vi "Analog Read N Chans.vi"(7 "Analog Ref Override":dbl, 8 "Error In":errorcluster, 10 "AI Channel(s)":u8[](array[numeric]), 11 "LINX Resource":T1) -> (0 "Error Out":errorcluster, 1 "AI Ref":dbl, 2 "Voltages":dbl[](array[numeric]), 3 "LINX Resource":T1)   [LabVIEW 2013, in "LVH-LINX.lvlib"]
doc: "Read the values of the specified analog input channels."
uses:
  <vilib>/LabVIEW Hacker/LINX/LVH-LINX.lvlib
  <vilib>/LabVIEW Hacker/LINX/Private/Type Defs/LINX Ref.ctl
  <vilib>/LabVIEW Hacker/LINX/Private/Type Defs/Platform.ctl
  <vilib>/LabVIEW Hacker/LINX/Private/Type Defs/Interface.ctl
  <vilib>/LabVIEW Hacker/LINX/Private/Device/Type Defs/LINX Device Config.ctl
  <vilib>/LabVIEW Hacker/LINX/Private/Device/Type Defs/TCP Config.ctl
  <vilib>/LabVIEW Hacker/LINX/Private/Type Defs/Device Family.ctl
  <vilib>/LabVIEW Hacker/LINX/Private/Type Defs/Peripheral.ctl
  <vilib>/LabVIEW Hacker/LINX/Private/Device/Device.lvlib
  <vilib>/LabVIEW Hacker/LINX/Private/myRIO/myRIO.lvlib
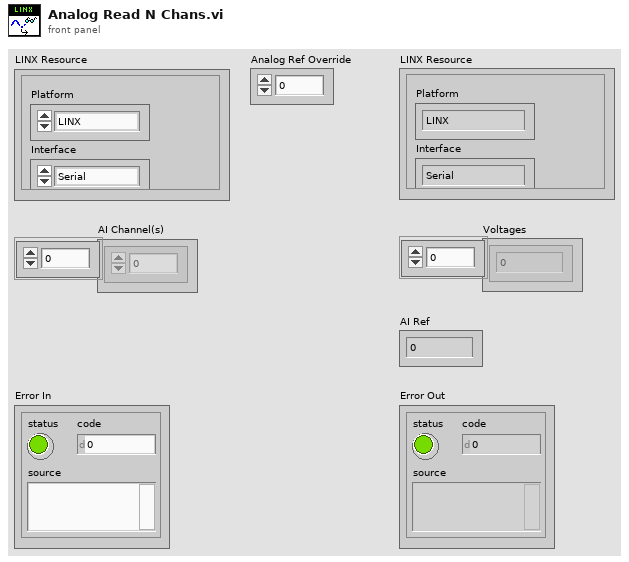
[diagram p1: front panel]
types:
  T1 = typedef "LVH-LINX.lvlib/LINX Ref.ctl" = cluster{"Platform":T2, "Interface":T3, "LINX Device Config":T4}
  T2 = typedef "LVH-LINX.lvlib/Platform.ctl" = enum16{"LINX", "myRIO"}
  T3 = typedef "LVH-LINX.lvlib/Interface.ctl" = enum16{"Serial", "TCP"}
  T4 = typedef "LVH-LINX.lvlib/Device.lvlib/LINX Device Config.ctl" = cluster{"Interface":T3, "COM Port":refnum<visa-resource-name>, "TCP Configuration":T5, "Device Family":T6, "Device ID":u8, "Device Name":string, "TCP Ref":refnum<k5>}
  T5 = typedef "LVH-LINX.lvlib/Device.lvlib/TCP Config.ctl" = cluster{"IP Address":string, "Port":u16}
  T6 = typedef "LVH-LINX.lvlib/Device Family.ctl" = enum8{"National Instruments", "Digilent", "Arduino"}
  T7 = typedef "LVH-LINX.lvlib/Peripheral.ctl" = enum8{"DI", "DO", "AI", "AO", "PWM", "QE", "UART", "I2C", "SPI", "CAN"}
  T8 = typedef "AI.lvlib/AI Reference.ctl" = cluster{"myRIO Reference":T9, "AI Channels List":T13, "AI Scaling Constants List":T15}
  T9 = typedef "myRIO Generic Hardware Reference.ctl" = cluster{"myRIO Model":T10, "myRIO Hardware Reference":T11}
  T10 = typedef "Hardware Version Enum.ctl" = enum16{"Unknown", "myRIO-1900", "myRIO-1950"}
  T11 = typedef "myRIO v1.0 Reference.ctl" = cluster{"Generic FPGA Reference":T12, "Allow multiple opens":bool}
  T12 = typedef "Generic FPGA Reference.ctl" = refnum<k20>
  T13 = typedef "AI Channels List.ctl" = T14[]
  T14 = typedef "AI Channels Enum.ctl" = enum16{"Not Connected", "AudioIn/Left", "AudioIn/Right", "C/AI0", "C/AI1", "A/AI0", "A/AI1", "A/AI2", "A/AI3", "B/AI0", "B/AI1", "B/AI2", "B/AI3"}
  T15 = typedef "Analog Scaling Constants List.ctl" = T16[]
  T16 = typedef "Analog Scaling Constants.ctl" = cluster{"LSB Weight (Volts)":dbl, "Offset (Volts)":dbl, "Signed?":bool}
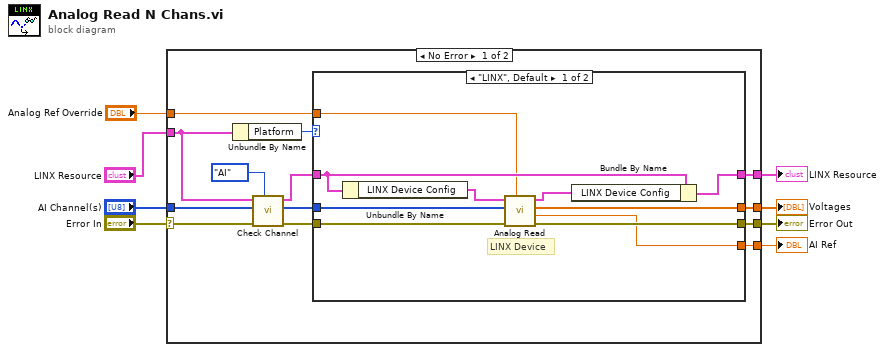
[diagram p0: block diagram]
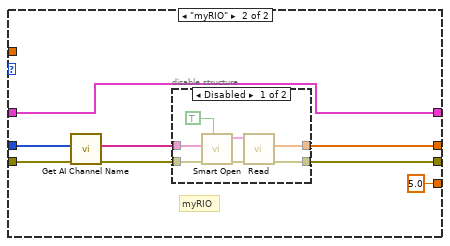
[diagram p2: hidden frame]
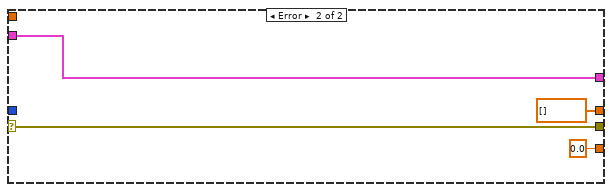
[diagram p4: hidden frame]
diagram:
  n1 = case shown="No Error" "Error In" {
    selector: "Error In" -> [w10 w51]
    tunnel: [w20 w51] -> w8
    tunnel: [w19 w49] -> w7
    tunnel: "LINX Resource" -> [w14 w49]
    tunnel: "AI Channel(s)" -> [w13 _]
    tunnel: [w12 dbl[] [] ("Values")] -> w4
    tunnel: "Analog Ref Override" -> [w11 _]
    tunnel: [w9 0.0 ("AI Ref")] -> w1
    frame No Error {
      n2 = Unbundle By Name(w14) -> ("Platform"=w21:T2)
      n3 = call <vilib>:"Check Channel.vi"("Peripheral"=Peripheral."AI", "Error In"=w10, "Channels"=w13, "LINX Resource"=w14) -> ("Error Out"=w18:errorcluster, "Channels"=w17:u8[], "LINX Resource"=w15:T1)  [unwired: 5 in]
      n4 = case shown="\"LINX\", Default" w21 {
        tunnel: w18 -> [w28 w34]
        tunnel: w15 -> [w31 w39]
        tunnel: [w29 w37] -> w20
        tunnel: [w30 w39] -> w19
        tunnel: w17 -> [w25 w38]
        tunnel: [w24 w35] -> w12
        tunnel: w11 -> [w23 _]
        tunnel: [w22 5.0 ("AI Ref")] -> w9
        frame "LINX", Default {
          # "LINX Device"
          n5 = Unbundle By Name(w31) -> ("LINX Device Config"=w27:T4)
          n6 = call <vilib>:"Analog Read.vi"("Analog Ref Override"=w23, "Error In"=w28, "AI Channels"=w25, "LINX Device Config"=w27) -> ("Error Out"=w29:errorcluster, "AI Ref"=w22:dbl, "Voltages"=w24:dbl[], "LINX Device Config"=w26:T4)  [unwired: 4 in]
          n7 = Bundle By Name(cluster=w31, "LINX Device Config"=w26) -> (w30:T1)
        }
        frame "myRIO" {
          # "myRIO"
          n8 = call <vilib>:"Get AI Channel Name.vi"("Error In"=w34, "AI Channel Nums"=w38) -> ("Error Out"=w33:errorcluster, "AI Channels"=w36:string[])  [unwired: 7 in]
          n9 = disable-structure shown="Disabled" {
            disable-tunnel: w33 -> [w44 w47]
            disable-tunnel: [w43 w47] -> w37
            disable-tunnel: w36 -> [w41 _]
            disable-tunnel: [w40 _] -> w35
            frame Disabled {
              n10 = call <vilib>:"Smart Open.vi"("Allow multiple opens?"=TRUE, "error in (no error)"=w44, "Channel Names"=w41) -> ("error out"=w46:errorcluster, "AI Ref Out"=w45:T8)  [unwired: 7 in]
              n11 = call <vilib>:"Read.vi"("error in (no error)"=w46, "AI Ref In"=w45) -> ("error out"=w43:errorcluster, "Values"=w40:dbl[])  [unwired: 7 in, 1 out]
            }
            frame Enabled {
              # "Thow myRIO\nSupport error"
            }
          }
        }
      }
    }
    frame Error {
    }
  }
  "Error Out" <- w8
  "LINX Resource" <- w7
  "Voltages" <- w4
  "AI Ref" <- w1
